vi "Spin Coater Low Level Write.vi"(7 "Solution ID":i32, 8 "Error In":errorcluster, 9 "Current Layer ID":i32, 10 "Layer Information Cluster":T2 {"Deposition Method" items=["Blade Coating", "Spin Coating", "Thermal Evaporation", "E-Beam Evaporation", "Sputtering", "Drop Casting", "Dip Coating", "Pulsed Laser Deposition", "Chemival Vapour Deposition", "Atomic Layer Deposition", "Spray Coating", "Screen Printing", "Electroplating", "Molecular Beam Epitaxy", "Custom Deposition"]; "Layer Type" items=["Front Electrode", "Electron Transport Layer", "Active Layer", "Hole Transport Layer", "Back Electrode", "Custom Layer"]}, 11 "Refnum in":T1) -> (0 "Error Out":errorcluster, 3 "Refnum out":T1)   [LabVIEW 2020]
uses:
  Data Clusters/Layer Information Cluster.ctl
  <vilib>/addons/database/Connection.llb/Conn ObjectReference.ctl
  <vilib>/addons/database/NI_Database_API.lvlib
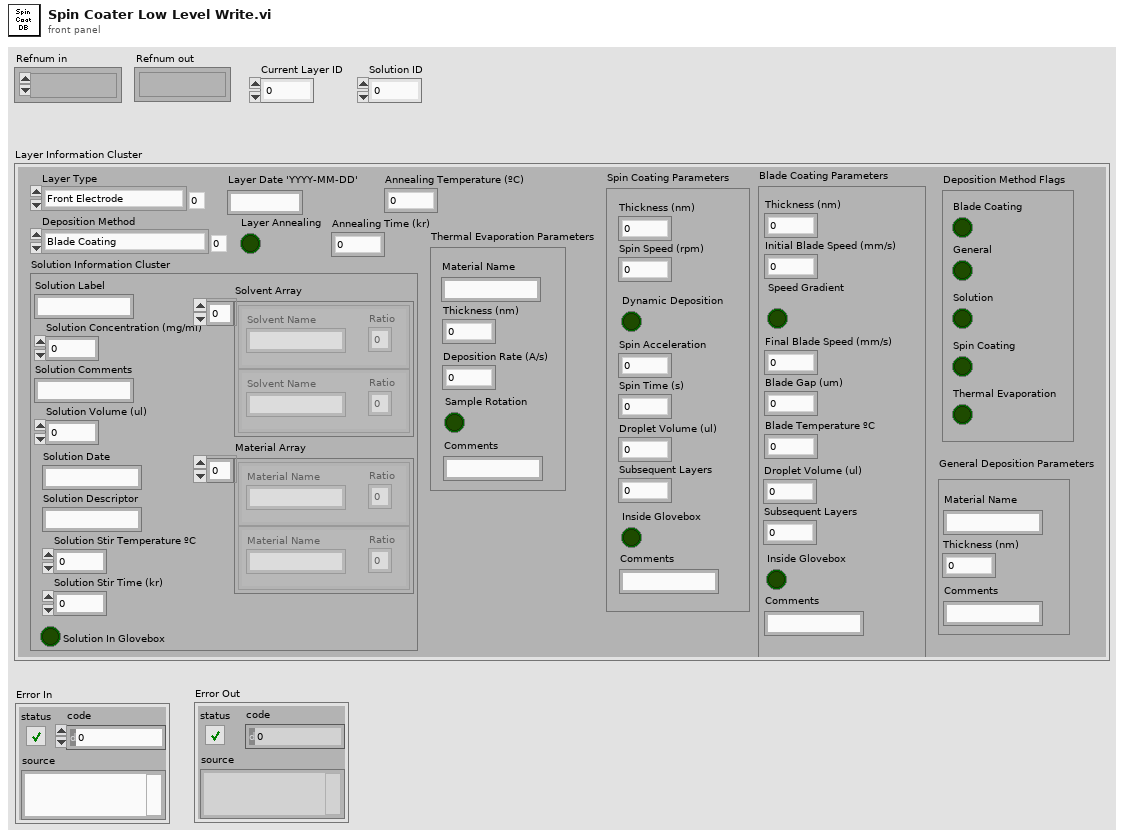
[diagram p1: front panel]
types:
  T1 = typedef "NI_Database_API.lvlib/Conn ObjectReference.ctl" = refnum<k1>
  T2 = typedef "Layer Information Cluster.ctl" = cluster{"Solution Information Cluster":cluster{"Solution Label":string, "Solution Concentration (mg/ml)":dbl, "Solution Comments ":string, "Solution Volume (ul) ":dbl, "Solution Date ":string, "Solution Descriptor ":string, "Solution Stir Temperature ºC ":dbl, "Solution Stir Time (kr) ":dbl, "Solution In Glovebox":bool, "Solvent Array":cluster{"Solvent Name":string, "Ratio":dbl}[], "Material Array":cluster{"Material Name":string, "Ratio":dbl}[]}, "Layer Type":u16, "Deposition Method":u16, "Layer Annealing":bool, "General Deposition Parameters":cluster{"Thickness (nm)":dbl, "Comments":string, "Material Name":string}, "Blade Coating Parameters":cluster{"Thickness (nm)":dbl, "Initial Blade Speed (mm/s)":dbl, "Speed Gradient":bool, "Final Blade Speed (mm/s)":dbl, "Blade Gap (um)":dbl, "Droplet Volume (ul)":dbl, "Subsequent Layers":dbl, "Inside Glovebox":bool, "Comments":string, "Blade Temperature ºC":dbl}, "Spin Coating Parameters":cluster{"Thickness (nm)":dbl, "Spin Speed (rpm)":dbl, "Dynamic Deposition":bool, "Spin Acceleration":dbl, "Spin Time (s)":dbl, "Droplet Volume (ul)":dbl, "Subsequent Layers":dbl, "Inside Glovebox":bool, "Comments":string}, "Thermal Evaporation Parameters":cluster{"Deposition Rate (A/s)":dbl, "Thickness (nm)":dbl, "Comments":string, "Material Name":string, "Sample Rotation":bool}, "Layer Date 'YYYY-MM-DD'":string, "Annealing Time (kr)":dbl, "Annealing Temperature (ºC)":dbl, "Deposition Method Flags":cluster{"Blade Coating":bool, "General ":bool, "Solution":bool, "Spin Coating":bool, "Thermal Evaporation":bool}}
  T3 = cluster{"Thickness (nm)":dbl, "Spin Speed (rpm)":dbl, "Dynamic Deposition":bool, "Spin Acceleration":dbl, "Spin Time (s)":dbl, "Droplet Volume (ul)":dbl, "Subsequent Layers":dbl, "Inside Glovebox":bool, "Comments":string, "Current Layer ID":i32}
  T4 = cluster{"Solution ID":i32, "Thickness (nm)":dbl, "Spin Speed (rpm)":dbl, "Dynamic Deposition":bool, "Spin Acceleration":dbl, "Spin Time (s)":dbl, "Droplet Volume (ul)":dbl, "Subsequent Layers":dbl, "Inside Glovebox":bool, "Comments":string, "Current Layer ID":i32}
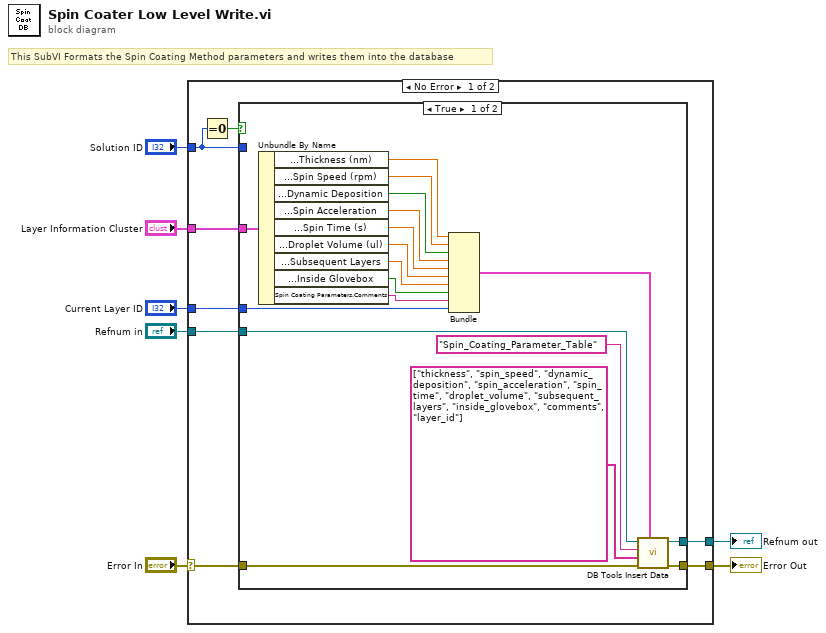
[diagram p0: block diagram]
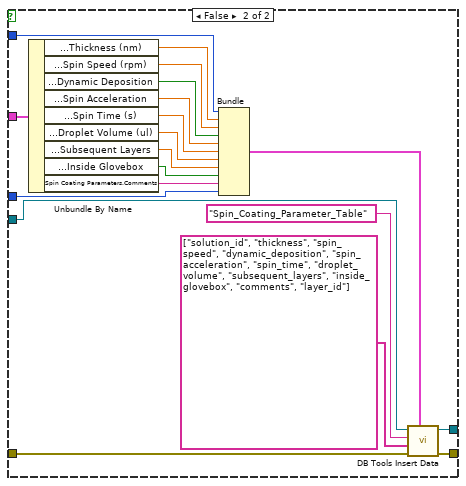
[diagram p2: hidden frame]
diagram:
  # "This SubVI Formats the Spin Coating Method parameters and writes them into the database"
  n1 = case shown="No Error" "Error In" {
    selector: "Error In" -> [w11 w53]
    tunnel: "Solution ID" -> [w15 _]
    tunnel: "Layer Information Cluster" -> [w13 _]
    tunnel: "Current Layer ID" -> [w12 _]
    tunnel: "Refnum in" -> [w10 w54]
    tunnel: [w9 w54] -> w2
    tunnel: [w8 w53] -> w1
    frame No Error {
      n2 = Equal To 0?(x=w15) -> (x = 0?=w14:bool)
      n3 = case shown="True" w14 {
        tunnel: [w33 w52] -> w8
        tunnel: [w32 w51] -> w9
        tunnel: w10 -> [w31 w50]
        tunnel: w11 -> [w30 w49]
        tunnel: w12 -> [w17 w37]
        tunnel: w13 -> [w29 w48]
        tunnel: w15 -> [_ w34]
        frame True {
          n4 = Unbundle By Name(w29) -> ("Spin Coating Parameters.Thickness (nm)"=w26:dbl, "Spin Coating Parameters.Spin Speed (rpm)"=w25:dbl, "Spin Coating Parameters.Dynamic Deposition"=w24:bool, "Spin Coating Parameters.Spin Acceleration"=w23:dbl, "Spin Coating Parameters.Spin Time (s)"=w22:dbl, "Spin Coating Parameters.Droplet Volume (ul)"=w21:dbl, "Spin Coating Parameters.Subsequent Layers"=w20:dbl, "Spin Coating Parameters.Inside Glovebox"=w19:bool, "Spin Coating Parameters.Comments"=w18:string)
          n5 = Bundle("Thickness (nm)"=w26, "Spin Speed (rpm)"=w25, "Dynamic Deposition"=w24, "Spin Acceleration"=w23, "Spin Time (s)"=w22, "Droplet Volume (ul)"=w21, "Subsequent Layers"=w20, "Inside Glovebox"=w19, "Comments"=w18, "Current Layer ID"=w17) -> (w16:T3)  [unwired: 1 in]
          n6 = call <vilib>:"DB Tools Insert Data.vi"("data"=w16, "error in (no error)"=w30, "columns"=string[] ["thickness", "spin_speed", "dynamic_deposition", "spin_acceleration", "spin_time", "droplet_volume", "subsequent_layers", "inside_glovebox", "comments", "layer_id"], "table"="Spin_Coating_Parameter_Table", "connection reference"=w31) -> ("error out"=w33:errorcluster, "connection reference out"=w32:T1)  [unwired: 5 in]
        }
        frame False {
          n7 = Unbundle By Name(w48) -> ("Spin Coating Parameters.Thickness (nm)"=w46:dbl, "Spin Coating Parameters.Spin Speed (rpm)"=w45:dbl, "Spin Coating Parameters.Dynamic Deposition"=w44:bool, "Spin Coating Parameters.Spin Acceleration"=w43:dbl, "Spin Coating Parameters.Spin Time (s)"=w42:dbl, "Spin Coating Parameters.Droplet Volume (ul)"=w41:dbl, "Spin Coating Parameters.Subsequent Layers"=w40:dbl, "Spin Coating Parameters.Inside Glovebox"=w39:bool, "Spin Coating Parameters.Comments"=w38:string)
          n8 = Bundle("Solution ID"=w34, "Thickness (nm)"=w46, "Spin Speed (rpm)"=w45, "Dynamic Deposition"=w44, "Spin Acceleration"=w43, "Spin Time (s)"=w42, "Droplet Volume (ul)"=w41, "Subsequent Layers"=w40, "Inside Glovebox"=w39, "Comments"=w38, "Current Layer ID"=w37) -> (w36:T4)  [unwired: 1 in]
          n9 = call <vilib>:"DB Tools Insert Data.vi"("data"=w36, "error in (no error)"=w49, "columns"=string[] ["solution_id", "thickness", "spin_speed", "dynamic_deposition", "spin_acceleration", "spin_time", "droplet_volume", "subsequent_layers", "inside_glovebox", "comments", "layer_id"], "table"="Spin_Coating_Parameter_Table", "connection reference"=w50) -> ("error out"=w52:errorcluster, "connection reference out"=w51:T1)  [unwired: 5 in]
        }
      }
    }
    frame Error {
    }
  }
  "Refnum out" <- w2
  "Error Out" <- w1
